vi "Build Stim Init Cmd.vi"(0 "Stimulator":T1={"Stim Open Data"={"Name"="", "Mode"=enum."LIVE", "Visa Timeout"=0}, "Stim Init Data"={"Frequency"=0.0, "N Factor"=0, "D/T Int"=0.0, "Active Channels"=[FALSE], "LF Channels"=[]}, "Stim Update Data"={"Pulse Mode"=[], "Current"=[], "Pulse Dur"=[]}, "Stim Status"={"Open"=FALSE, "On"=FALSE}}) -> (2 "Stimulator":T1={"Stim Open Data"={"Name"="", "Mode"=enum."LIVE", "Visa Timeout"=0}, "Stim Init Data"={"Frequency"=0.0, "N Factor"=0, "D/T Int"=0.0, "Active Channels"=[FALSE], "LF Channels"=[]}, "Stim Update Data"={"Pulse Mode"=[], "Current"=[], "Pulse Dur"=[]}, "Stim Status"={"Open"=FALSE, "On"=FALSE}}, 3 "Command":T7)   [LabVIEW 2019]
uses:
  Data Type Defs/Stimulator.ctl
  Data Type Defs/Stim Open Data.ctl
  Data Type Defs/Stim Init Data.ctl
  Data Type Defs/Stim Update Data.ctl
  Data Type Defs/Pulse Mode (array).ctl
  Data Type Defs/Stim Status.ctl
  NumArray to CatStr.vi
  Archive/StrArray to CatStr.vi
panel:
  out "N-Factor":u8
  out "Interpulse Interval (ms)":dbl
  out "Channel LF Boolean Array":bool[](array[boolean])
  out "Channel Stim Boolean Array":bool[](array[boolean])=[TRUE, TRUE, TRUE, TRUE, TRUE]
  out "Stim Frequency (Hz)":dbl=40.0
  # "Inputs\nStim Frequency - the main frequency of stimulation in Hz.  The Hasomed Rehastim Science Mode documentation defines this as 1/t1.  We typically use 40 Hz for FES applications.\nGroup Time - for multi-pulse stimulation, enter the inter-pulse interval (aka pulse repetition interval) here.  We typically use single pulses (Group Time = 0).\nN factor - the factor by which t1 is multiplied to get the \"Low Frequency\" channel period.  This is optional - we typically do not use it.\nChannel Stim Boolean Array - defines the active channels (up to 8).\nChannel LF Boolean Array - defines the channels for which \"low frequency\" will be used.  Low frequency is defined as 1/(N_factor * Stim_Frequency).\n\nOutputs\nChannel List Mode Init Cmd String - the string of Hex numbers representing the final command."
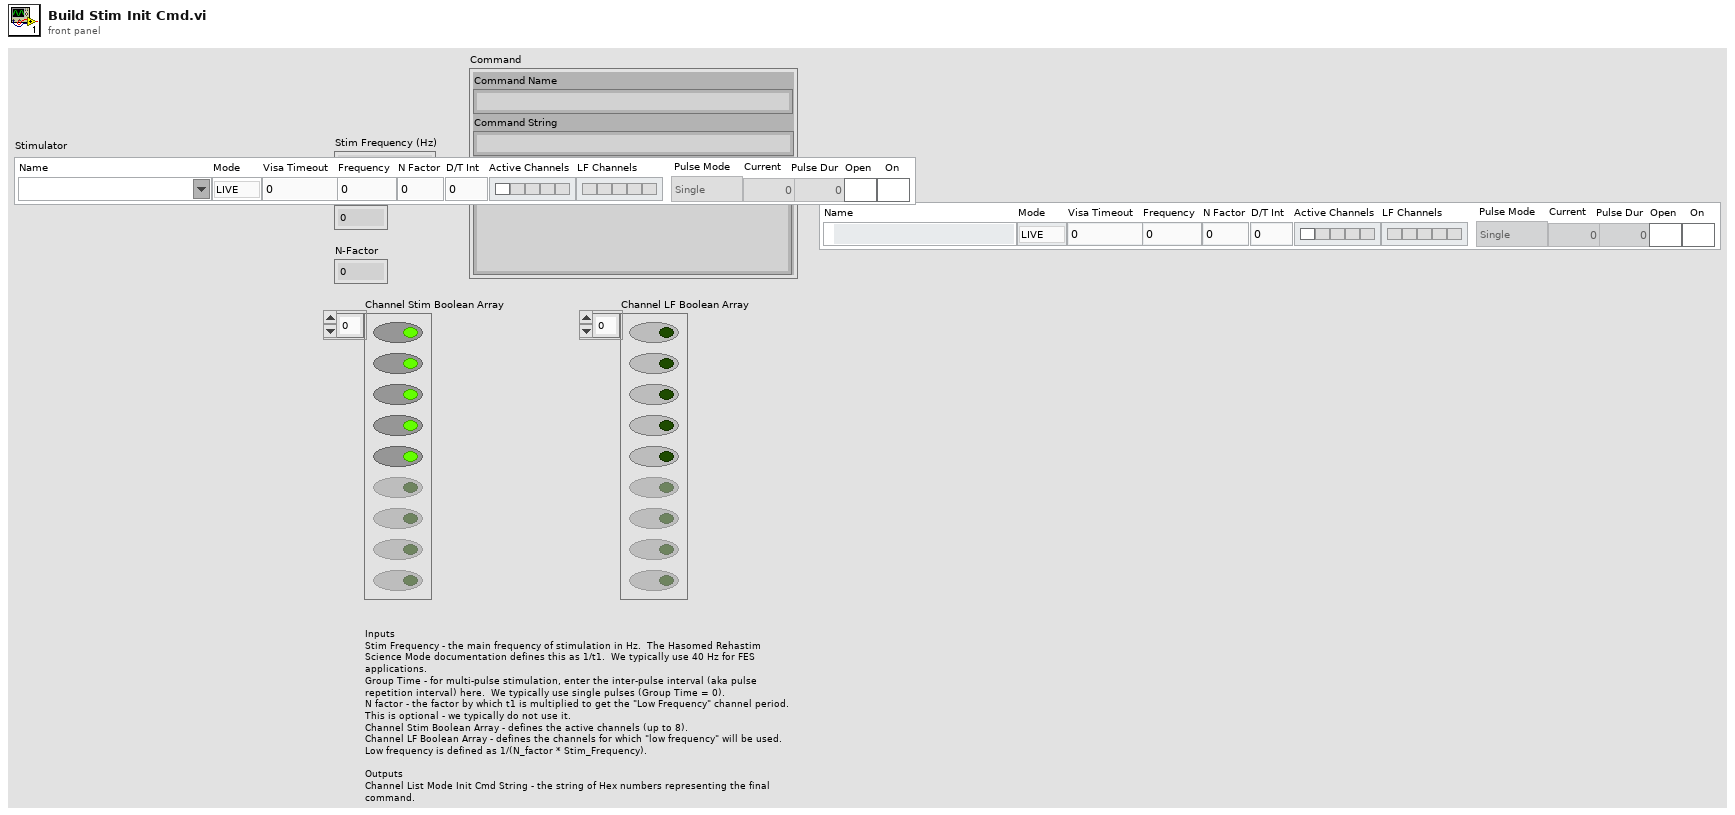
[diagram p1: front panel]
types:
  T1 = typedef "Stimulator.ctl" = cluster{"Stim Open Data":T2, "Stim Init Data":T3, "Stim Update Data":T4, "Stim Status":T6}
  T2 = typedef "Stim Open Data.ctl" = cluster{"Name":refnum<visa-resource-name>, "Mode":enum16{"LIVE", "SIM"}, "Visa Timeout":u32}
  T3 = typedef "Stim Init Data.ctl" = cluster{"Frequency":dbl, "N Factor":u8, "D/T Int":dbl, "Active Channels":bool[], "LF Channels":bool[]}
  T4 = typedef "Stim Update Data.ctl" = cluster{"Pulse Mode":T5, "Current":u32[], "Pulse Dur":u32[]}
  T5 = typedef "Pulse Mode (array).ctl" = enum16{"Single", "Doublet", "Triplet"}[]
  T6 = typedef "Stim Status.ctl" = cluster{"Open":bool, "On":bool}
  T7 = cluster{"Command Name":string, "Command String":string, "Log String":string}
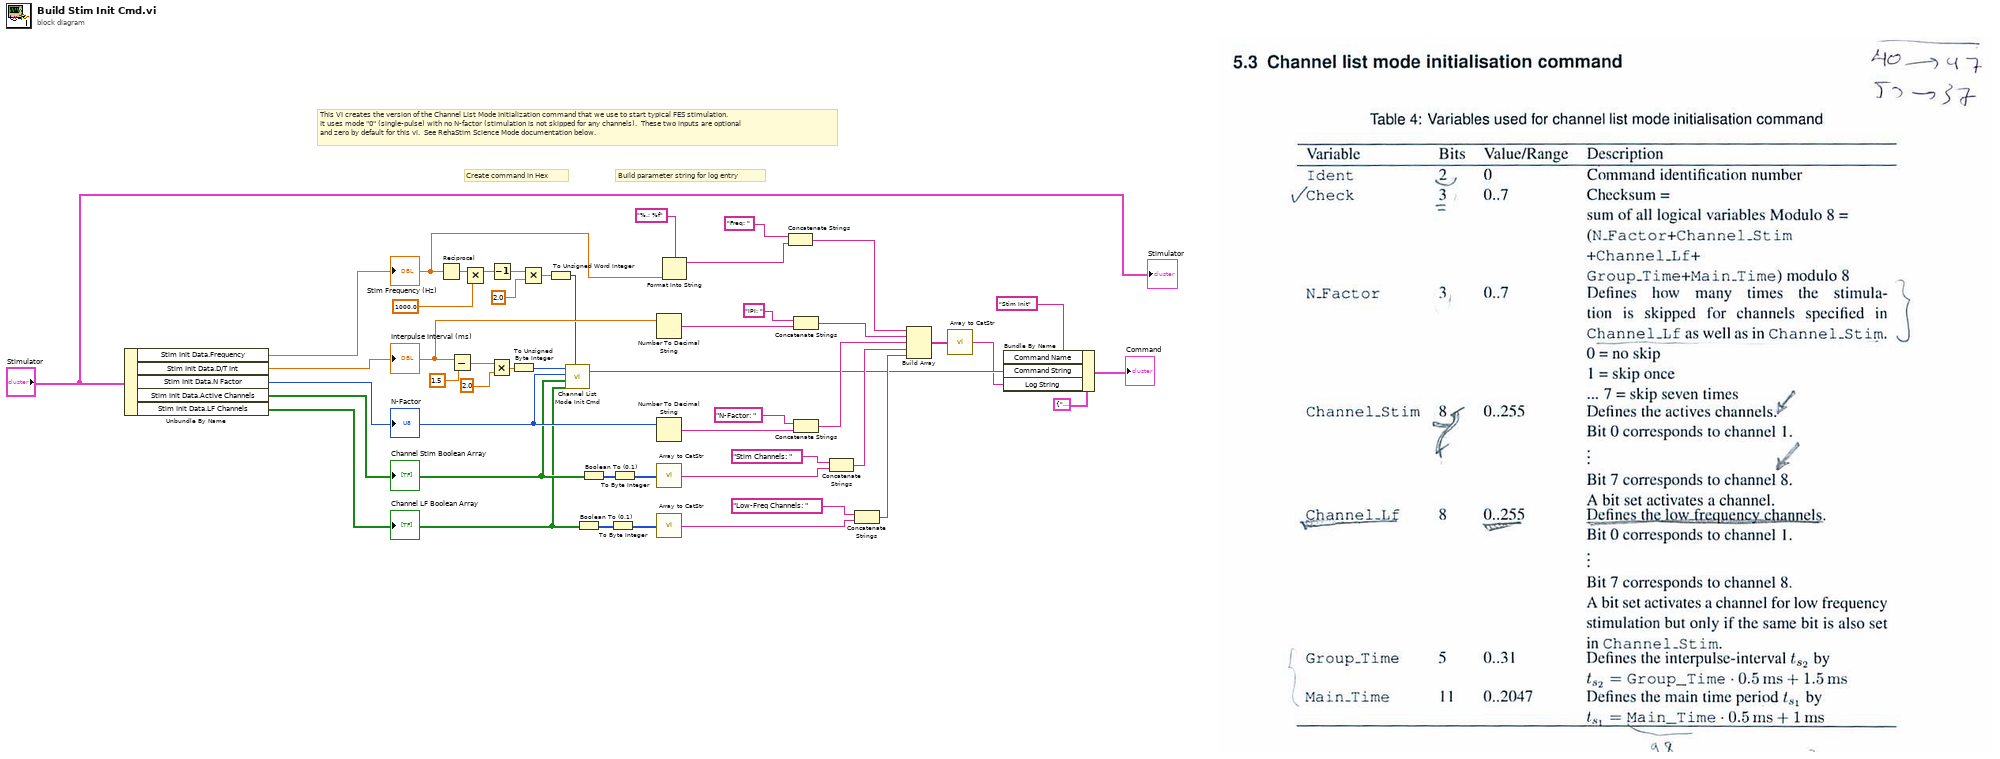
[diagram p0: block diagram]
diagram:
  # "Build parameter string for log entry"
  # "Create command in Hex"
  # "This VI creates the version of the Channel List Mode Initialization command that we use to start typical FES stimulation.\nIt uses mode \"0\" (single-pulse) with no N-factor (stimulation is not skipped for any channels).  These two inputs are optional\nand zero by default for this vi.  See RehaStim Science Mode documentation below."
  n1 = Unbundle By Name("Stimulator") -> ("Stim Init Data.Frequency"=w11:dbl, "Stim Init Data.D/T Int"=w15:dbl, "Stim Init Data.N Factor"=w14:u8, "Stim Init Data.Active Channels"=w13:bool[], "Stim Init Data.LF Channels"=w12:bool[])
  "Stim Frequency (Hz)" <- w11
  "Channel Stim Boolean Array" <- w13
  "Channel LF Boolean Array" <- w12
  "Interpulse Interval (ms)" <- w15
  "N-Factor" <- w14
  n2 = Reciprocal(x=w11) -> (1/x=w44:dbl)
  n3 = Subtract(x=w15, y=1.5) -> (x-y=w38:dbl)
  n4 = Multiply(x=w44, y=1000.0) -> (x*y=w41:dbl)
  n5 = Multiply(x=w38, y=2.0) -> (x*y=w36:dbl)
  n6 = Decrement(x=w41) -> (x-1=w43:dbl)
  n7 = To Unsigned Byte Integer(number=w36) -> (unsigned 8bit integer=w2:u8)
  n8 = Multiply(x=w43, y=2.0) -> (x*y=w35:dbl)
  n9 = To Unsigned Word Integer(number=w35) -> (unsigned 16bit integer=w3:u16)
  n10 = call "Channel List Mode Init Cmd.vi"("Main time"=w3, "Channel LF Boolean Array"=w12, "Channel Stim Boolean Array"=w13, "N factor"=w14, "Group Time"=w2) -> ("Channel List Mode Init Cmd String"=w6:string)  [unwired: 2 in]
  n11 = Boolean To (0,1)(Boolean=w12) -> (0, 1=w31:i16[])
  n12 = Boolean To (0,1)(Boolean=w13) -> (0, 1=w33:i16[])
  n13 = To Byte Integer(number=w31) -> (8bit integer=w30:i8[])
  n14 = To Byte Integer(number=w33) -> (8bit integer=w32:i8[])
  n15 = Number To Decimal String(number=w15) -> (decimal integer string=w26:string)  [unwired: 1 in]
  n16 = Number To Decimal String(number=w14) -> (decimal integer string=w23:string)  [unwired: 1 in]
  n17 = call-poly "Array to CatStr.vi"("Array"=w32) -> ("spreadsheet string"=w21:string)
  n18 = call-poly "Array to CatStr.vi"("Array"=w30) -> ("spreadsheet string"=w19:string)
  n19 = Format Into String(format string="%.; %f", w11) -> (resulting string=w9:string)  [unwired: 2 in, 1 out]
  n20 = Concatenate Strings("Freq: " ("string"), w9) -> (w28:string)
  n21 = Concatenate Strings("IPI: " ("string"), w26) -> (w25:string)
  n22 = Concatenate Strings("N-Factor: " ("string"), w23) -> (w18:string)
  n23 = Concatenate Strings("Stim Channels: " ("string"), w21) -> (w17:string)
  n24 = Concatenate Strings("Low-Freq Channels: " ("string"), w19) -> (w16:string)
  n25 = Build Array(w28, w25, w18, w17, w16) -> (w34:string[])
  n26 = call-poly "Array to CatStr.vi"("String Array"=w34) -> ("spreadsheet string"=w5:string)
  n27 = Bundle By Name(cluster=T7 {"Command Name"="", "Command String"="", "Log String"=""}, "Command Name"="Stim Init", "Command String"=w6, "Log String"=w5) -> (→"Command":T7)
  "Stimulator" <- "Stimulator"
